vi "runscenario get reports.vi"(8 "error in (no error)":errorcluster, 11 "jobid":string) -> (0 "error out":errorcluster, 1 "READY?":bool, 3 "Datasheet Paths":T1[](array[typedef]))   [LabVIEW 2011]
uses:
  server/DIAdem/Datasheet/Datasheet Report Info.ctl
  Summitek EXT/OpenG EXT/file/file.llb/File Exists - Scalar__ogtk.vi
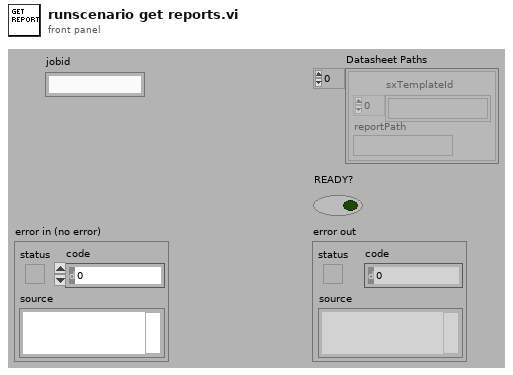
[diagram p1: front panel]
types:
  T1 = typedef "Datasheet Report Info.ctl" = cluster{"sxTemplateId":string[], "reportPath":path}
  T2 = typedef "DATASHEET Report Info.ctl" = cluster{"sxTemplateId":string[], "reportPath":path}
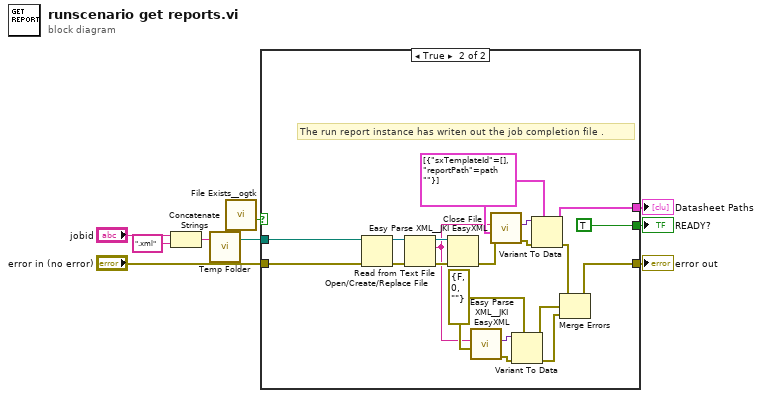
[diagram p0: block diagram]
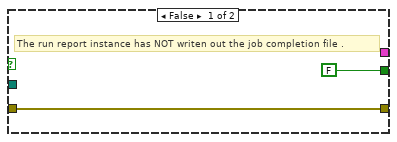
[diagram p2: hidden frame]
diagram:
  n1 = Concatenate Strings("jobid", ".xml" ("string")) -> (w8:string)
  n2 = call "Temp Folder.vi"("Relative Path (\"\")"=w8) -> ("Temp Folder"=w2:path)  [unwired: 2 in]
  n3 = call-poly "File Exists__ogtk.vi"("file path"=w2) -> ("exists"=w3:bool)  [unwired: 6 in, 1 out]
  n4 = case shown="True" w3 {
    tunnel: [FALSE ("READY?") TRUE ("READY?")] -> w9
    tunnel: [w10 w14] -> w5
    tunnel: w2 -> [_ w26]
    tunnel: [_ w21] -> w4
    tunnel: "error in (no error)" -> [w10 w20]
    frame False {
      # "The run report instance has NOT writen out the job completion file ."
    }
    frame True {
      w18 = errorcluster {"status"=FALSE, "code"=0, "source"=""} ("error out")
      w23 = T2[] [{"sxTemplateId"=[], "reportPath"=path ""}] ("Datasheet Paths")
      # "The run report instance has writen out the job completion file ."
      n5 = Open/Create/Replace File(file path (use dialog)=w26, error in=w20) -> (refnum out=w27:refnum<file>, error out=w30:errorcluster)  [unwired: 4 in, 1 out]
      n6 = Read from Text File(file (use dialog)=w27, error in=w30) -> (refnum out=w28:refnum<file>, text=w16:string, error out=w29:errorcluster)  [unwired: 2 in, 1 out]
      n7 = Close File(refnum=w28, error in=w29) -> (error out=w25:errorcluster)  [unwired: 1 out]
      n8 = call "Easy Parse XML__JKI EasyXML.vi"("LabVIEW Data (Type)"=w18, "XML String"=w16) -> ("error out"=w17:errorcluster, "LabVIEW Data"=w19:variant)  [unwired: 8 in]
      n9 = call "Easy Parse XML__JKI EasyXML.vi"("error in (no error)"=w25, "LabVIEW Data (Type)"=w23, "XML String"=w16) -> ("error out"=w24:errorcluster, "LabVIEW Data"=w22:variant)  [unwired: 7 in]
      n10 = Variant To Data(error in=w17, type=w18, Variant=w19) -> (data=w13:errorcluster, error out=w12:errorcluster)
      n11 = Variant To Data(error in=w24, type=w23, Variant=w22) -> (data=w21:T2[], error out=w15:errorcluster)
      n12 = Merge Errors(w15, w13, w12) -> (w14:errorcluster)
    }
  }
  "error out" <- w5
  "READY?" <- w9
  "Datasheet Paths" <- w4
